vi "AH2500.RST.vi"(8 "error in (no error)":errorcluster, 11 "VISA resource name":refnum<visa-resource-name>) -> (0 "error out":errorcluster, 1 "Read string":string="UC= 9456.092   PF L= 658.76     NS V=0.10   V\r\n", 2 "Send string":string="UNITS 1;\nSHOW UN", 3 "VISA resource name out":refnum<visa-resource-name>)   [LabVIEW 2019, in "Inst.AH2500.lvclass"]
uses:
  Inst.AH2500.lvclass
panel:
  # "RESET"
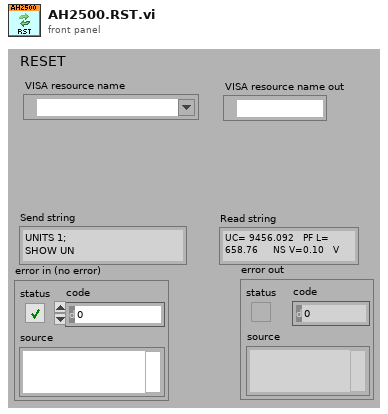
[diagram p1: front panel]
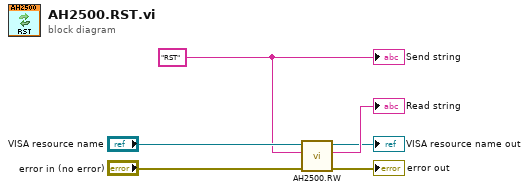
[diagram p0: block diagram]
diagram:
  w1 = "RST" ("format string")
  n1 = call "AH2500.RW.vi"("error in (no error)"="error in (no error)", "write buffer"=w1, "VISA Refnum in"="VISA resource name") -> ("error out"=→"error out":errorcluster, "read buffer"=→"Read string":string, "VISA Refnum out"=→"VISA resource name out":refnum<visa-resource-name>)  [unwired: 6 in]
  "Send string" <- w1
